vi "CAENHV Set Ch Param Bitfield.vi"(5 "ParValue":bool[](array[boolean]), 6 "ChList":u16[](array[numeric]), 7 "ChNum":u16, 8 "error in (no error)":errorcluster, 9 "ParName":string, 10 "slot":u16, 11 "handle":i32) -> (0 "error out":errorcluster)   [LabVIEW 2009, in "CAENHVWrapper.lvlib"]
doc: "CAENHVLIB_API CAENHVRESULT CAENHV_SetChParam(int handle, ushort slot, \n const char *ParName, ushort ChNum, const ushort *ChList, void *ParValue);"
uses:
  <userlib>/CAENHVWrapper/CAENHVWrapper.lvlib
  <userlib>/CAENHVWrapper/CAENHVWrapper.dll
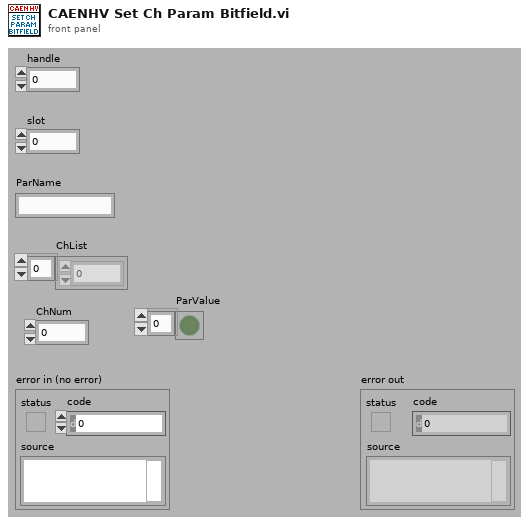
[diagram p1: front panel]
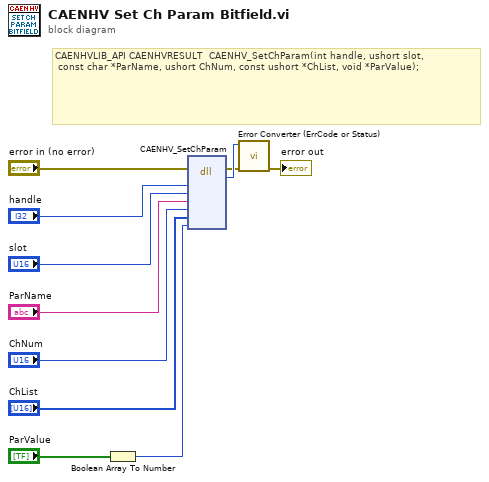
[diagram p0: block diagram]
diagram:
  # "CAENHVLIB_API CAENHVRESULT  CAENHV_SetChParam(int handle, ushort slot, \n const char *ParName, ushort ChNum, const ushort *ChList, void *ParValue);"
  n1 = Boolean Array To Number(Boolean array="ParValue") -> (number=w1:u32)
  n2 = dll-call lib="C:/Program Files/National Instruments/LabVIEW 2009/user.lib/CAENHVWrapper/CAENHVWrapper.*" fn="CAENHV_SetChParam"(error in="error in (no error)", "handle"="handle", "slot"="slot", "ParName"="ParName", "ChNum"="ChNum", "ChList"="ChList", "ParValue"=w1) -> (error out=w5:errorcluster, "return type"=w6:i32)  [unwired: 8 in, 1 out]
  n3 = call <userlib>:"Error Converter (ErrCode or Status).vi"("error in (no error)"=w5, "error code"=w6) -> ("error out"=→"error out":errorcluster)  [unwired: 9 in]
